vi "convertChannels.vi"(8 "error in (no error)":errorcluster, 11 "HamegHMPSupply in":refnum<class "HamegHMPSupply.lvclass">) -> (0 "error out":errorcluster, 2 "channels":i32[](array[numeric]), 3 "HamegHMPSupply out":refnum<class "HamegHMPSupply.lvclass">)   [LabVIEW 2011, in "Hardware.lvlib" / "Channels.lvlib" / "HamegHMPSupply.lvclass"]
uses:
  HamegHMPSupply.lvclass
  HamegHMPSupply.lvclass/HamegHMPSupply.ctl
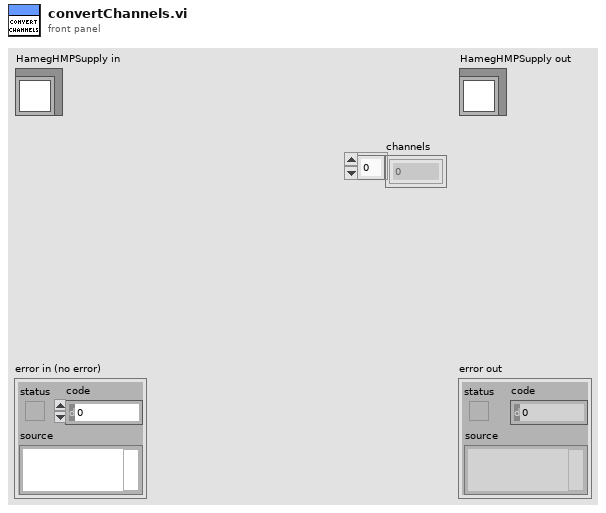
[diagram p1: front panel]
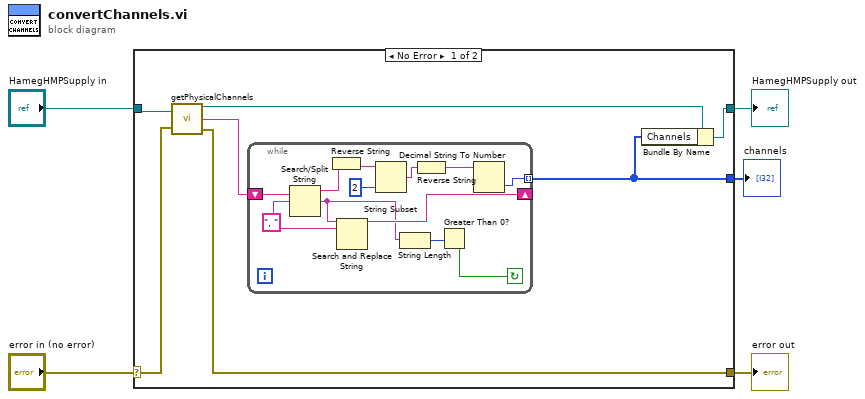
[diagram p0: block diagram]
diagram:
  n1 = case shown="No Error" "error in (no error)" {
    selector: "error in (no error)" -> [w11 w26]
    tunnel: [w7 w26] -> w4
    tunnel: [w8 w25] -> w2
    tunnel: "HamegHMPSupply in" -> [w12 w25]
    tunnel: [w6 _] -> w1
    frame No Error {
      n2 = call-dynamic "getPhysicalChannels.vi"("AnalogOutput.lvclass in"=w12, "error in (no error)"=w11) -> ("AnalogOutput.lvclass out"=w9:refnum<class "HamegHMPSupply.lvclass">, "Physical Channels"=w10:string, "error out"=w7:errorcluster)
      n3 = while {
        shift-right: [w22] -> _
        shift-left: w10 -> [w24]
        tunnel: [w16] -> w6 mode=indexing
        stop <- w13 continue-if-true
        w23 = ", "
        n4 = Search/Split String(string=w24, search string/char (-)=w23) -> (substring before match=w21:string, match + rest of string=w14:string)  [unwired: 1 in, 1 out]
        n5 = Reverse String(1:w21) -> (0:w20:string)
        n6 = Search and Replace String(input string=w14, search string=w23) -> (result string=w22:string)  [unwired: 6 in, 3 out]
        n7 = String Subset(string=w20, length (rest)=2) -> (substring=w18:string)  [unwired: 1 in]
        n8 = String Length(string=w14) -> (length=w15:i32)
        n9 = Reverse String(1:w18) -> (0:w17:string)
        n10 = Greater Than 0?(x=w15) -> (x > 0?=w13:bool)
        n11 = Decimal String To Number(string=w17) -> (number=w16:i32)  [unwired: 2 in, 1 out]
      }
      n12 = Bundle By Name(cluster=w9, "Channels"=w6) -> (w8:refnum<class "HamegHMPSupply.lvclass">)
    }
    frame Error {
    }
  }
  "error out" <- w4
  "HamegHMPSupply out" <- w2
  "channels" <- w1
